vi "isEXE.vi"(8 "Error In":errorcluster) -> (0 "Error Out":errorcluster, 3 "Boolean":bool)   [LabVIEW 2018]
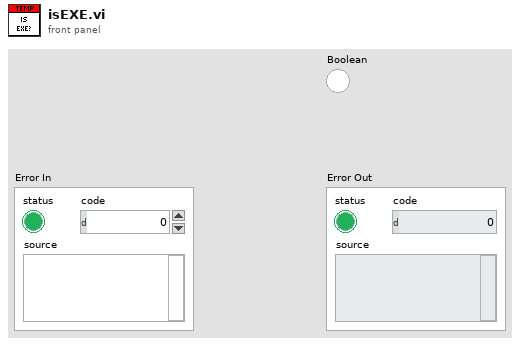
[diagram p1: front panel]
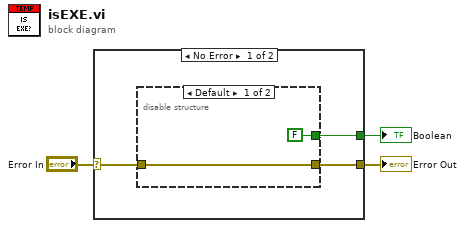
[diagram p0: block diagram]
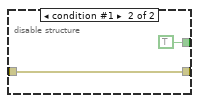
[diagram p2: hidden frame]
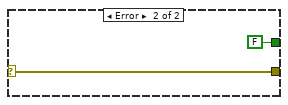
[diagram p3: hidden frame]
diagram:
  n1 = case shown="No Error" "Error In" {
    selector: "Error In" -> [w6 w12]
    tunnel: [w5 w12] -> w2
    tunnel: [w4 FALSE] -> w1
    frame No Error {
      n2 = disable-structure shown="Default" {
        disable-tunnel: w6 -> [w8 w10]
        disable-tunnel: [w8 w10] -> w5
        disable-tunnel: [FALSE TRUE] -> w4
        frame condition #0 (active) {
        }
        frame condition #1 {
        }
      }
    }
    frame Error {
    }
  }
  "Error Out" <- w2
  "Boolean" <- w1
